vi "XL320_Read Applied Torque.vi"(8 "error in (no error)":errorcluster, 10 "Motor ID (0)":u8, 11 "VISA resource name":refnum<visa-resource-name>) -> (0 "error out":errorcluster, 2 "Load/torque %":sgl, 3 "VISA resource name out":refnum<visa-resource-name>)   [LabVIEW 2017, in "Dynamixel XL320.lvlib"]
doc: "Retrieves the value for the amound of torque the motor is applying."
uses:
  <instrlib>/Dynamixel XL320 (Drivers instrument)/Dynamixel XL320.lvlib
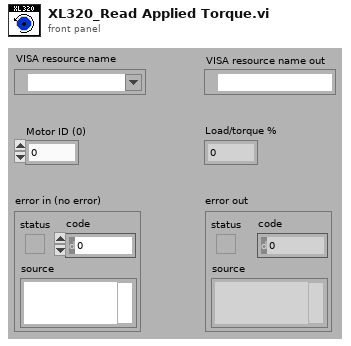
[diagram p1: front panel]
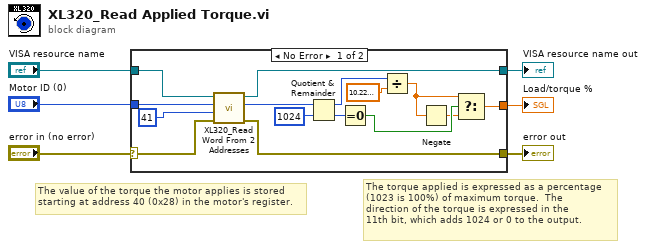
[diagram p0: block diagram]
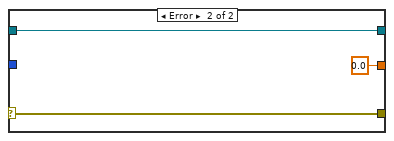
[diagram p2: hidden frame]
diagram:
  # "The torque applied is expressed as a percentage\n(1023 is 100%) of maximum torque.  The\ndirection of the torque is expressed in the \n11th bit, which adds 1024 or 0 to the output."
  # "The value of the torque the motor applies is stored\nstarting at address 40 (0x28) in the motor's register."
  n1 = case shown="No Error" "error in (no error)" {
    selector: "error in (no error)" -> [w10 w23]
    tunnel: [w17 sgl 0.0] -> w6
    tunnel: [w7 w23] -> w5
    tunnel: "VISA resource name" -> [w13 w24]
    tunnel: [w9 w24] -> w3
    tunnel: "Motor ID (0)" -> [w12 _]
    frame No Error {
      n2 = call <instrlib>:"XL320_Read Word From 2 Addresses.vi"("Error in (no error)"=w10, "Address number (0)"=u16 41 ("Address # DEC"), "Motor ID (0)"=w12, "VISA resource name"=w13) -> ("error out"=w7:errorcluster, "Data"=w8:u16, "VISA resource name out"=w9:refnum<visa-resource-name>)  [unwired: 5 in]
      n3 = Quotient & Remainder(x=w8, y=1024) -> (x-y*floor(x/y)=w16:i32, floor(x/y)=w20:i32)
      n4 = Equal To 0?(x=w20) -> (x = 0?=w19:bool)
      n5 = Divide(x=w16, y=sgl 10.23) -> (x/y=w14:sgl)
      n6 = Negate(x=w14) -> (-x=w18:sgl)
      n7 = Select(t=w14, s=w19, f=w18) -> (s? t:f=w17:sgl)
    }
    frame Error {
    }
  }
  "VISA resource name out" <- w3
  "error out" <- w5
  "Load/torque %" <- w6
